vi "9219_Initialize.vi"(8 "error in (no error)":errorcluster, 9 "Slot Settings":T1, 11 "9219 in":refnum<class "9219.lvclass">) -> (0 "error out":errorcluster, 3 "9219 out":refnum<class "9219.lvclass">)   [LabVIEW 2020, in "Modules.lvlib" / "9219.lvclass"]
uses:
  9219.lvclass
  RSI Module/Slot Settings.ctl
  C:/Users/nitest/Desktop/Git 2020/niveristand-scan-engine-module-libraries/Source/RSI Module/RSI Module.lvclass
  RSI Module/Channels.ctl
  RSI Module/Channel Type.ctl
  RSI Module/Module Models.ctl
  9219.lvclass/9219.ctl
  RSI Module/RSI Module.lvclass
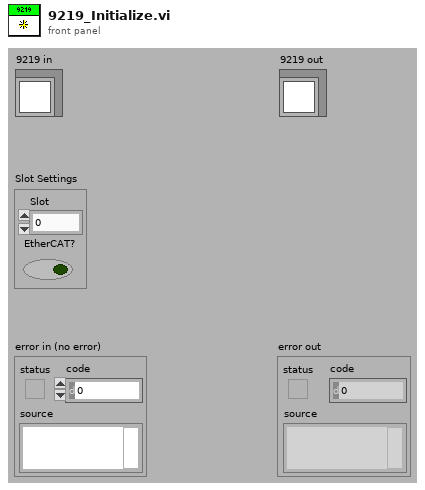
[diagram p1: front panel]
types:
  T1 = typedef "Modules.lvlib/RSI Module.lvclass/Slot Settings.ctl" = cluster{"Slot":u32, "EtherCAT?":bool}
  T2 = typedef "Modules.lvlib/RSI Module.lvclass/Module Models.ctl" = enum16{"Empty", "NI 9201", "NI 9203", "NI 9205", "NI 9206", "NI 9207", "NI 9208", "NI 9209", "NI 9210", "NI 9211", "NI 9212", "NI 9213", "NI 9214", "NI 9215", "NI 9216", "NI 9217", "NI 9219", "NI 9220", "NI 9221", "NI 9222", "NI 9223", "NI 9224", "NI 9225", "NI 9226", "NI 9227", "NI 9228", "NI 9229", "NI 9233", "NI 9234", "NI 9235", "NI 9236", "NI 9237", "NI 9239", "NI 9242", "NI 9244", "NI 9253", "NI 9263", "NI 9264", "NI 9265", "NI 9266", "NI 9269", "NI 9344", "NI 9350", "NI 9375", "NI 9401", "NI 9402", "NI 9403", "NI 9411", "NI 9421", "NI 9422", "NI 9423", "NI 9425", "NI 9426", "NI 9435", "NI 9436", "NI 9437", "NI 9472", "NI 9474", "NI 9475", "NI 9476", "NI 9477", "NI 9478", "NI 9481", "NI 9482", "NI 9485"}
  T3 = cluster{"Degree range":u32, "Digital threshold":dbl, "Range / Mode":u32, "RTD type":u32, "RTD A":dbl, "RTD B":dbl, "RTD C":dbl, "RTD Ro":dbl, "Thermocouple type":u32}
  T4 = typedef "Modules.lvlib/RSI Module.lvclass/Channels.ctl" = cluster{"# Input Channels":i32, "# Output Channels":i32, "Channel Type":T5, "Units":string}
  T5 = typedef "Modules.lvlib/RSI Module.lvclass/Channel Type.ctl" = enum16{"Analog", "Digital"}
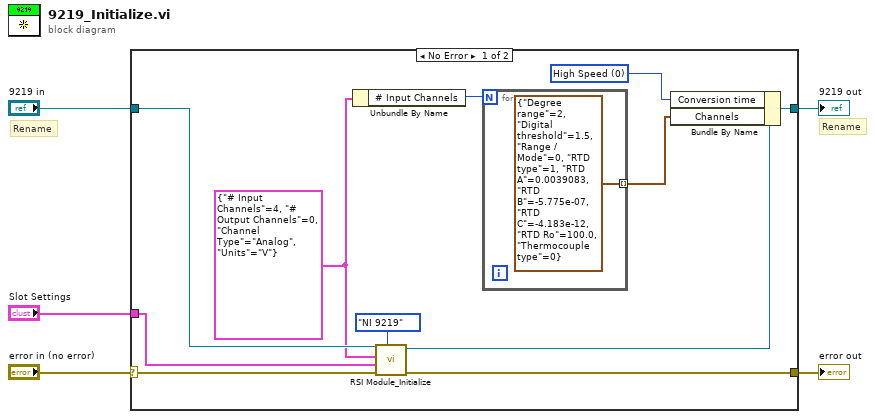
[diagram p0: block diagram]
diagram:
  # "Rename"
  # "Rename"
  n1 = case shown="No Error" "error in (no error)" {
    selector: "error in (no error)" -> [w14 w19]
    tunnel: [w13 w19] -> w4
    tunnel: [w11 w18] -> w2
    tunnel: "9219 in" -> [w16 w18]
    tunnel: "Slot Settings" -> [w15 _]
    frame No Error {
      w6 = u32 0 items=["High Speed", "60 Hz Reject", "50 Hz Reject", "High Resolution"] ("Conversion time")
      w9 = T4 {"# Input Channels"=4, "# Output Channels"=0, "Channel Type"=enum."Analog", "Units"="V"} ("Channels")
      n2 = Unbundle By Name(w9) -> ("# Input Channels"=w8:i32)
      n3 = call "RSI Module_Initialize.vi"("Module Model"=Module_Models."NI 9219", "error in (no error)"=w14, "Slot Settings"=w15, "Channels"=w9, "RSI Module in"=w16) -> ("error out"=w13:errorcluster, "RSI Module out"=w12:refnum<class "9219.lvclass">)  [unwired: 5 in]
      n4 = for {
        N: w8 -> [_]
        tunnel: [T3 {"Degree range"=2, "Digital threshold"=1.5, "Range / Mode"=0, "RTD type"=1, "RTD A"=0.0039083, "RTD B"=-5.775e-07, "RTD C"=-4.183e-12, "RTD Ro"=100.0, "Thermocouple type"=0} ("Channel")] -> w7 mode=indexing
      }
      n5 = Bundle By Name(cluster=w12, "Conversion time"=w6, "Channels"=w7) -> (w11:refnum<class "9219.lvclass">)
    }
    frame Error {
    }
  }
  "error out" <- w4
  "9219 out" <- w2
